vi "save control values.vi"(5 "Append timestamp (true)":bool=TRUE, 6 "error in":errorcluster, 8 "Dont save":string[](array[string]), 9 "Path":path) -> (0 "error out":errorcluster, 3 "file path out":path)   [LabVIEW 2020, in "POLARIS Vision utility.lvlib"]
doc: "from ni.com \nauthor mmiers."
uses:
  POLARIS Vision utility.lvlib
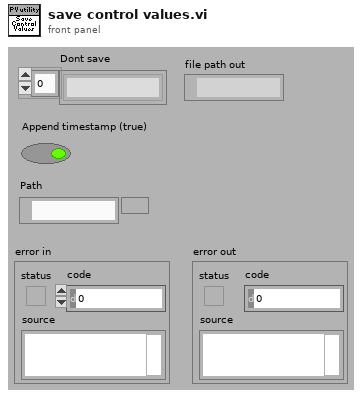
[diagram p1: front panel]
types:
  T1 = cluster{"Name":string, "type string":i16[], "data string":string}[]
  T2 = enum32{"invalid app kind", "Development System", "Run Time System", "Student Edition", "Embedded LabVIEW", "Evaluation", "Custom"}
  T3 = cluster{"Name":string, "type string":i16[], "data string":string}
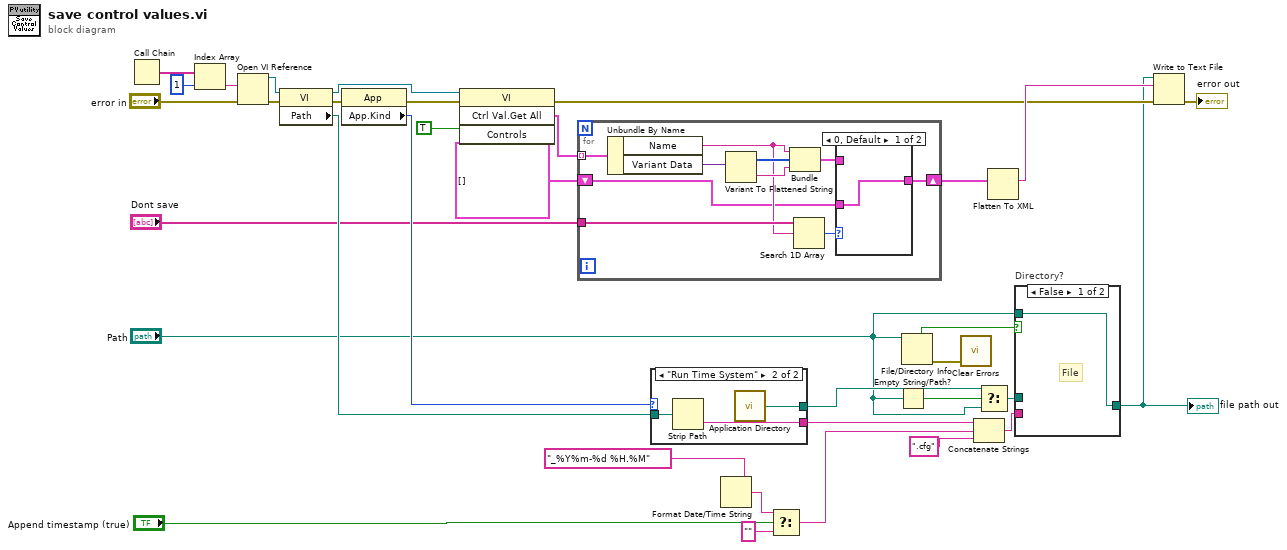
[diagram p0: block diagram]
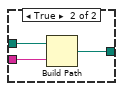
[diagram p2: hidden frame]
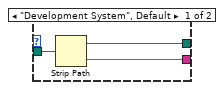
[diagram p3: hidden frame]
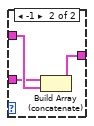
[diagram p4: hidden frame]
diagram:
  n1 = Call Chain() -> (call chain=w29:string[])
  n2 = Index Array(array=w29, index=1) -> (element=w25:string)
  n3 = Open VI Reference(vi path=w25, error in (no error)="error in") -> (vi reference=w24:refnum<vi>, error out=w26:errorcluster)  [unwired: 4 in]
  n4 = property class="VI"(reference=w24, error in=w26) -> (reference out=w4:refnum<vi>, error out=w21:errorcluster, "Path"=w23:path)
  n5 = property class="App"(error in=w21) -> (error out=w20:errorcluster, "App.Kind"=w22:T2)  [unwired: 1 in, 1 out]
  n6 = invoke class="VI" method="Ctrl Val.Get All"(reference=w4, error in=w20, "Controls"=TRUE ("Save control values")) -> (error out=w31:errorcluster, "Get All Control Values Variant"=w2:cluster{"Name":string, "Variant Data":variant}[])  [unwired: 1 in, 2 out]
  n7 = for {
    tunnel: w2 -> [w41] mode=indexing
    tunnel: "Dont save" -> [w40]
    shift-right: [w36] -> w32
    shift-left: T1 [] -> [w35]
    n8 = Unbundle By Name(w41) -> ("Name"=w39:string, "Variant Data"=w44:variant)
    n9 = Variant To Flattened String(Variant=w44) -> (data string=w42:string, 1:w43:i16[])
    n10 = Bundle("Name"=w39, "type string"=w43, "data string"=w42) -> (w37:T3)  [unwired: 1 out]
    n11 = Search 1D Array(1D array=w40, element=w39) -> (index of element=w38:i32)  [unwired: 1 in]
    n12 = case shown="0, Default" w38 {
      tunnel: w37 -> [_ w48]
      tunnel: [w45 w47] -> w36
      tunnel: w35 -> [w45 w46]
      frame 0, Default {
      }
      frame -1 {
        n13 = Build Array (concatenate)(w46, w48) -> (w47:T1)
      }
    }
  }
  n14 = case shown="\"Run Time System\"" w22 {
    tunnel: w23 -> [w51 w54]
    tunnel: [w50 w53] -> w10
    tunnel: [w49 w52] -> w15
    frame "Development System", Default {
      n15 = Strip Path(path=w51) -> (stripped path=w50:path, name=w49:string)
    }
    frame "Run Time System" {
      n16 = Strip Path(path=w54) -> (name=w52:string)  [unwired: 1 out]
      n17 = call <vilib>:"Application Directory.vi"() -> ("Application Directory"=w53:path)
    }
  }
  n18 = Format Date/Time String(time format string (%c)="_%Y%m-%d %H.%M") -> (date/time string=w13:string)  [unwired: 2 in]
  n19 = Select(t=w13, s="Append timestamp (true)", f="") -> (s? t:f=w12:string)
  n20 = Empty String/Path?(string/path="Path") -> (empty?=w9:bool)
  n21 = File/Directory Info(path="Path") -> (directory=w7:bool, error out=w5:errorcluster)  [unwired: 1 in, 5 out]
  n22 = call <vilib>:"Clear Errors.vi"("error in (no error)"=w5) -> ()  [unwired: 5 in, 2 out]
  n23 = Concatenate Strings(w15, w12, ".cfg" ("string")) -> (w18:string)
  n24 = Select(t=w10, s=w9, f="Path") -> (s? t:f=w8:path)
  n25 = Flatten To XML(6:w32) -> (2:w33:string)
  n26 = case "Directory?" shown="False" w7 {
    tunnel: [w55 w58] -> w19
    tunnel: w18 -> [_ w57]
    tunnel: w8 -> [_ w56]
    tunnel: "Path" -> [w55 _]
    frame False {
      # "File"
    }
    frame True {
      n27 = Build Path(base path=w56, name or relative path=w57) -> (appended path=w58:path)
    }
  }
  "file path out" <- w19
  n28 = Write to Text File(file (use dialog)=w19, text=w33, error in=w31) -> (error out=→"error out":errorcluster)  [unwired: 3 out]
